vi "AssertRunVI.vi"() -> ()   [LabVIEW 2016, in "DronaTest.lvlib"]
uses:
  DronaTest.lvlib
  APIs/Stimulus/VI/CloseVI.vi
  APIs/Stimulus/VI/RunVI.vi
  APIs/Assert/AssertVI/AssertVIExecRunning.vi
  <vilib>/addons/_JKI Toolkits/Caraya/classes/Assert/Assert Error.vi
  <vilib>/addons/_JKI Toolkits/Caraya/classes/Assert/Assert.lvclass
  <vilib>/addons/_JKI Toolkits/Caraya/classes/Test/Test.lvclass
  Drona.lvlib
  APIs/Stimulus/VI/VI.lvlib
  APIs/Assert/AssertVI/AssertVI.lvlib
panel:
  out "error out":errorcluster
  in  "error in":errorcluster
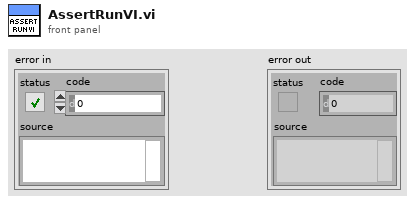
[diagram p1: front panel]
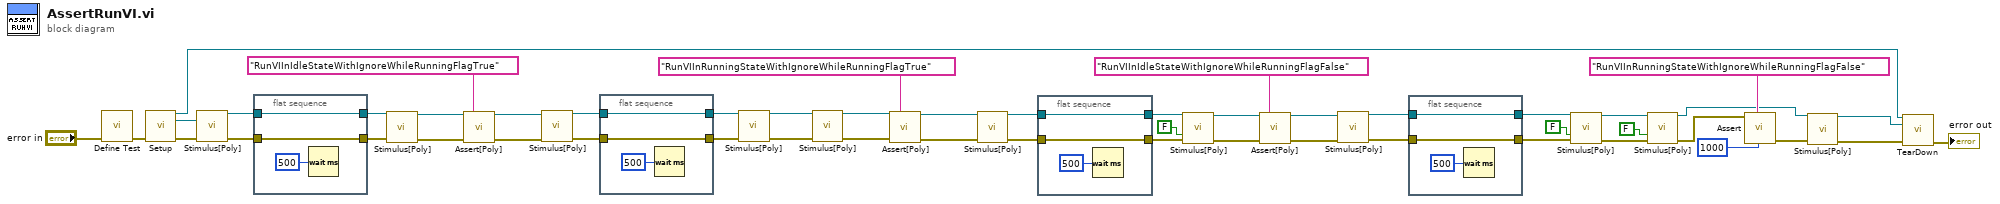
[diagram p0: block diagram]
diagram:
  n1 = call <vilib>:"Define Test.vi"("error in (no error)"="error in") -> ("error out"=w51:errorcluster)  [unwired: 9 in, 1 out]
  n2 = call "Setup.vi"("error in (no error)"=w51) -> ("Application Ref"=w2:refnum<vi>, "VI out"=w49:refnum<vi>, "error out"=w48:errorcluster)  [unwired: 12 in]
  n3 = call-poly "Stimulus[Poly].vi"("VI Reference In"=w49, "error in"=w48) -> ("VI Reference Out"=w23:refnum<vi>, "error out"=w22:errorcluster)  [unwired: 12 in]
  n4 = flat-sequence {
    tunnel: w23 -> [w53]
    tunnel: w22 -> [w54]
    tunnel: [w54] -> w21
    tunnel: [w53] -> w20
    frame #0 {
      n5 = Wait (ms)(milliseconds to wait=u32 500) -> ()  [unwired: 1 out]
    }
  }
  n6 = call-poly "Stimulus[Poly].vi"("VI Reference In"=w20, "error in"=w21) -> ("VI Reference Out"=w25:refnum<vi>, "error out"=w26:errorcluster)  [unwired: 12 in]
  n7 = call-poly "Assert[Poly].vi"("VI Reference In"=w25, "Test Label"="RunVIInIdleStateWithIgnoreWhileRunningFlagTrue", "Error In"=w26) -> ("VI Reference Out"=w27:refnum<vi>, "Error Out"=w28:errorcluster)  [unwired: 10 in, 1 out]
  n8 = call-poly "Stimulus[Poly].vi"("VI Reference In"=w27, "error in"=w28) -> ("VI Reference Out"=w18:refnum<vi>, "error out"=w19:errorcluster)  [unwired: 12 in]
  n9 = flat-sequence {
    tunnel: w18 -> [w56]
    tunnel: w19 -> [w57]
    tunnel: [w57] -> w16
    tunnel: [w56] -> w17
    frame #0 {
      n10 = Wait (ms)(milliseconds to wait=u32 500) -> ()  [unwired: 1 out]
    }
  }
  n11 = call-poly "Stimulus[Poly].vi"("VI Reference In"=w17, "error in"=w16) -> ("VI Reference Out"=w46:refnum<vi>, "error out"=w47:errorcluster)  [unwired: 12 in]
  n12 = call-poly "Stimulus[Poly].vi"("VI Reference In"=w46, "error in"=w47) -> ("VI Reference Out"=w45:refnum<vi>, "error out"=w44:errorcluster)  [unwired: 12 in]
  n13 = call-poly "Assert[Poly].vi"("VI Reference In"=w45, "Test Label"="RunVIInRunningStateWithIgnoreWhileRunningFlagTrue", "Error In"=w44) -> ("VI Reference Out"=w43:refnum<vi>, "Error Out"=w42:errorcluster)  [unwired: 10 in, 1 out]
  n14 = call-poly "Stimulus[Poly].vi"("VI Reference In"=w43, "error in"=w42) -> ("VI Reference Out"=w15:refnum<vi>, "error out"=w14:errorcluster)  [unwired: 12 in]
  n15 = flat-sequence {
    tunnel: w15 -> [w59]
    tunnel: w14 -> [w60]
    tunnel: [w60] -> w12
    tunnel: [w59] -> w13
    frame #0 {
      n16 = Wait (ms)(milliseconds to wait=u32 500) -> ()  [unwired: 1 out]
    }
  }
  n17 = call-poly "Stimulus[Poly].vi"("VI Reference In"=w13, "Ignore If Already Running (T)"=FALSE, "error in"=w12) -> ("VI Reference Out"=w40:refnum<vi>, "error out"=w39:errorcluster)  [unwired: 11 in]
  n18 = call-poly "Assert[Poly].vi"("VI Reference In"=w40, "Test Label"="RunVIInIdleStateWithIgnoreWhileRunningFlagFalse", "Error In"=w39) -> ("VI Reference Out"=w38:refnum<vi>, "Error Out"=w37:errorcluster)  [unwired: 10 in, 1 out]
  n19 = call-poly "Stimulus[Poly].vi"("VI Reference In"=w38, "error in"=w37) -> ("VI Reference Out"=w9:refnum<vi>, "error out"=w7:errorcluster)  [unwired: 12 in]
  n20 = flat-sequence {
    tunnel: w9 -> [w62]
    tunnel: w7 -> [w63]
    tunnel: [w63] -> w6
    tunnel: [w62] -> w8
    frame #0 {
      n21 = Wait (ms)(milliseconds to wait=u32 500) -> ()  [unwired: 1 out]
    }
  }
  n22 = call-poly "Stimulus[Poly].vi"("VI Reference In"=w8, "Ignore If Already Running (T)"=FALSE, "error in"=w6) -> ("VI Reference Out"=w36:refnum<vi>, "error out"=w35:errorcluster)  [unwired: 11 in]
  n23 = call-poly "Stimulus[Poly].vi"("VI Reference In"=w36, "Ignore If Already Running (T)"=FALSE, "error in"=w35) -> ("VI Reference Out"=w10:refnum<vi>, "error out"=w33:errorcluster)  [unwired: 11 in]
  n24 = call-poly <vilib>:"Assert.vi"("error code (1)"=1000, "Label"="RunVIInRunningStateWithIgnoreWhileRunningFlagFalse" ("Test Label"), "Error?"=w33) -> ("error out"=w11:errorcluster)  [unwired: 7 in, 1 out]
  n25 = call-poly "Stimulus[Poly].vi"("VI Reference In"=w10, "error in"=w11) -> ("VI Reference Out"=w4:refnum<vi>, "error out"=w5:errorcluster)  [unwired: 12 in]
  n26 = call "TearDown.vi"("Application Ref"=w2, "VI in"=w4, "error in (no error)"=w5) -> ("error out"=→"error out":errorcluster)  [unwired: 12 in]
